vi "CRYReport Pic TX LIB.vi"(6 "Control Ref":refnum<k7>, 7 "sAction":string, 8 "nData":i32, 9 "sData":string, 10 "TXTextControl":refnum<k7>, 11 "cFrame":T1) -> (0 "nData_Out":i32, 1 "sData_Out":string, 3 "cFrame_Out":T1)   [LabVIEW 2013]
uses:
  CRYReport Global.vi
  CRYProject/CRYProject Editor Global.vi
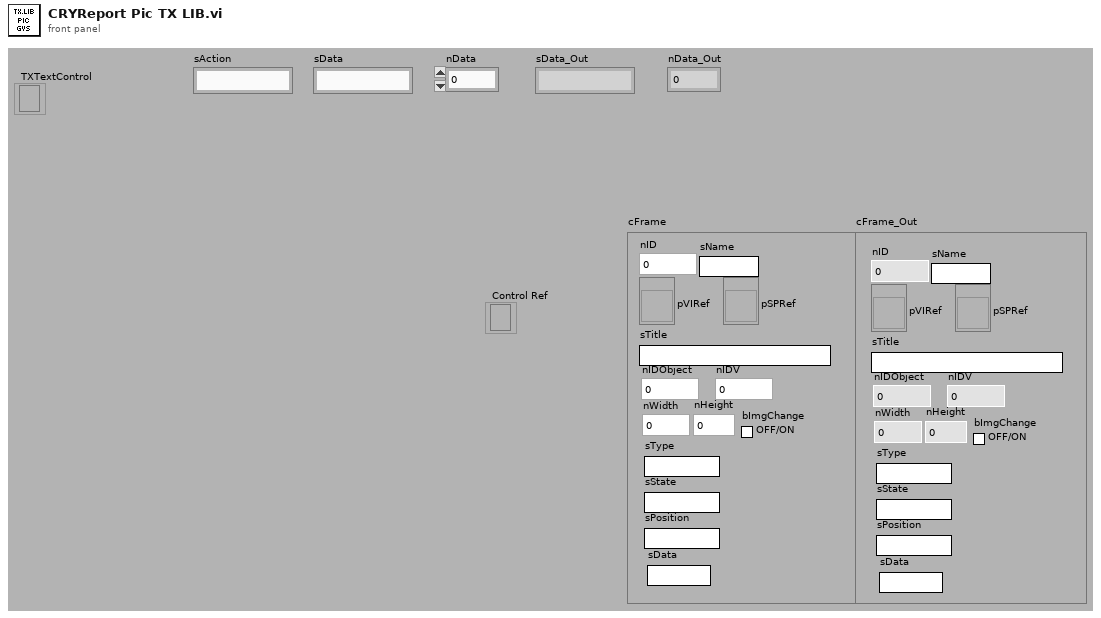
[diagram p1: front panel]
types:
  T1 = cluster{"nID":i16, "sName":string, "pVIRef":refnum<vi>, "pSPRef":refnum<vi>, "sTitle":string, "nIDObject":i16, "nIDV":i16, "nWidth":i16, "nHeight":i16, "bImgChange":bool, "sType":string, "sState":string, "sPosition":string, "sData":string}
  T2 = enum16{"open", "open or create", "create or replace", "create", "open (read only)"}
  T3 = typedef "CRYTS.ctl" = cluster{"No.TS":u16, "TS File Path":path, "TS Name":string, "EditStepName":string, "Steps":T4[], "New State":bool, "Change State":bool, "Flattened CurveLib Data":string, "Document Data":string, "EditStepNo":u16, "Operator Start File":string, "Sequence Type":string, "Sequence Language":string}
  T4 = typedef "CRYStep.ctl" = cluster{"No.VI":i32, "Category":string, "StepName":string, "Seq setup flattened":string, "Comment":string, "Steps config.":bool[], "Jump config":i32[], "Start":dbl, "Increment":dbl, "Name":string, "Unit":string, "Y data":u16, "Y prefix":string, "Y dB ref":dbl, "Y unit":string, "Repeat State Array":cluster{"Start":dbl, "Increment":dbl, "Count":i32, "Num":i32}[]}
  T5 = typedef "LVRectTypeDef.ctl" = cluster{"Left":i16, "Top":i16, "Right":i16, "Bottom":i16}
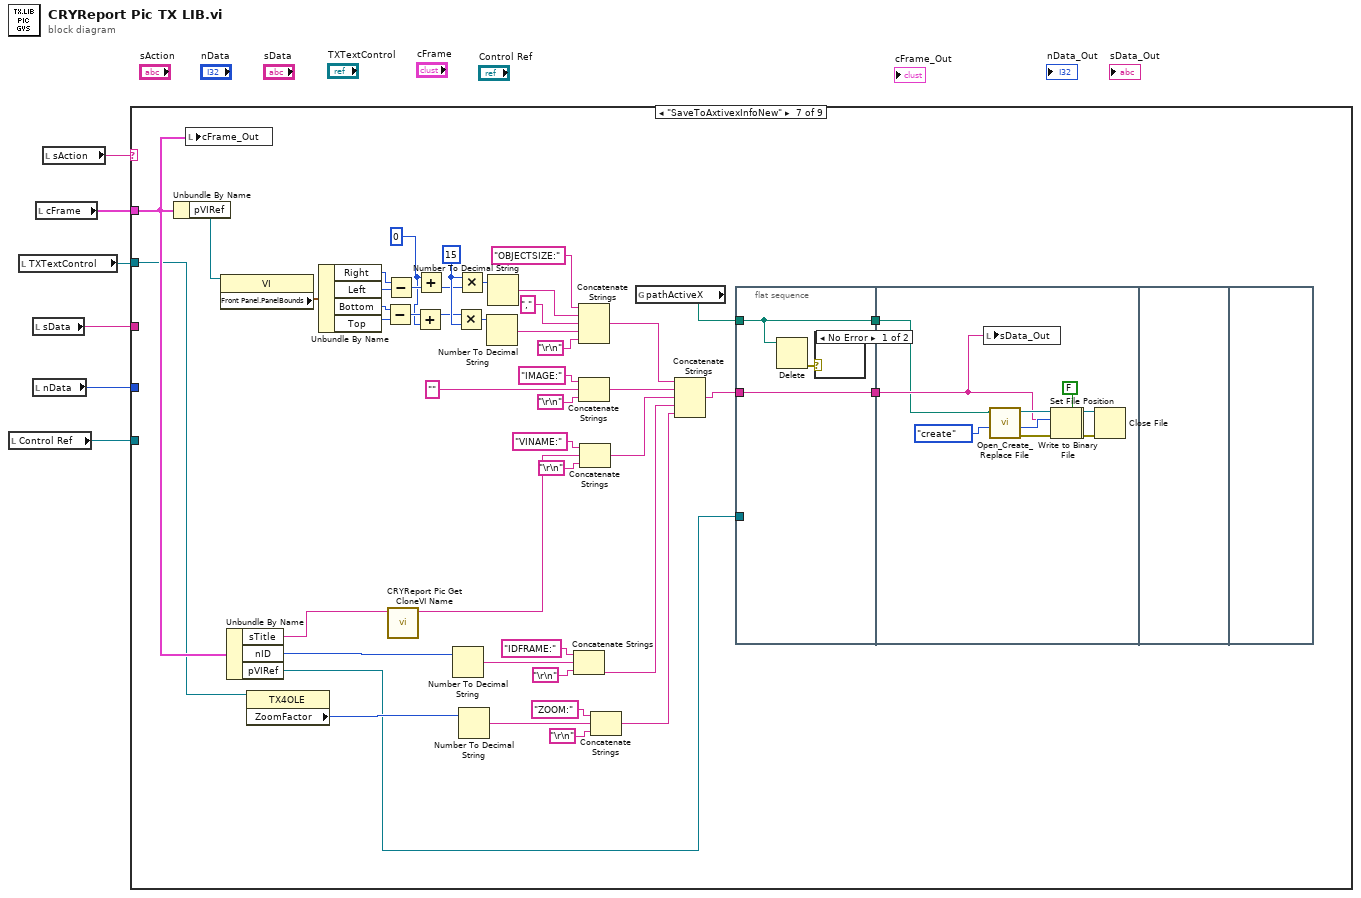
[diagram p0: block diagram]
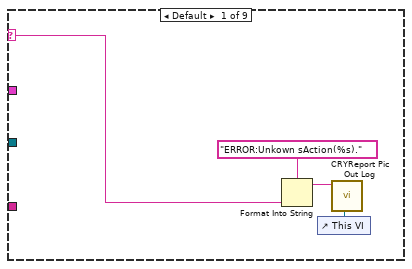
[diagram p2: hidden frame]
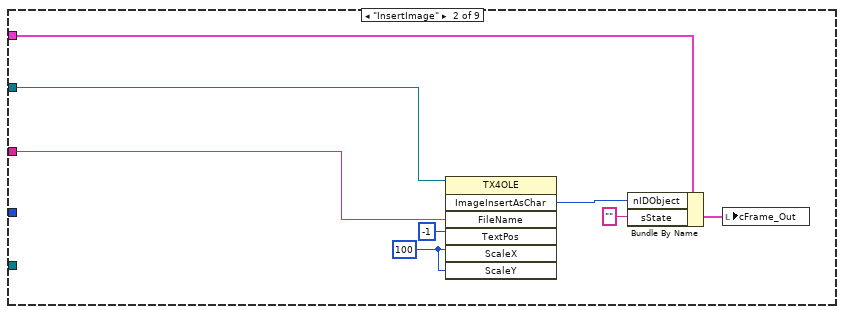
[diagram p3: hidden frame]
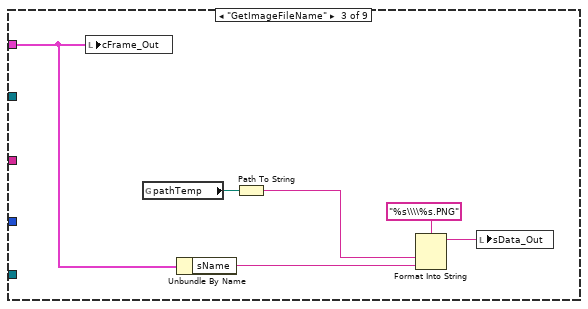
[diagram p4: hidden frame]
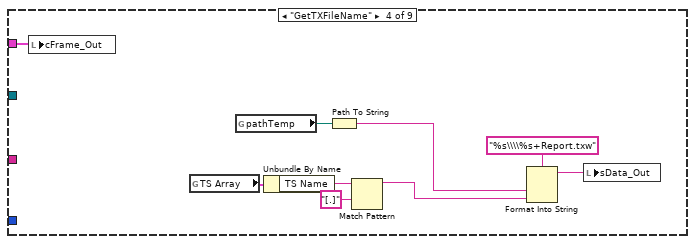
[diagram p5: hidden frame]
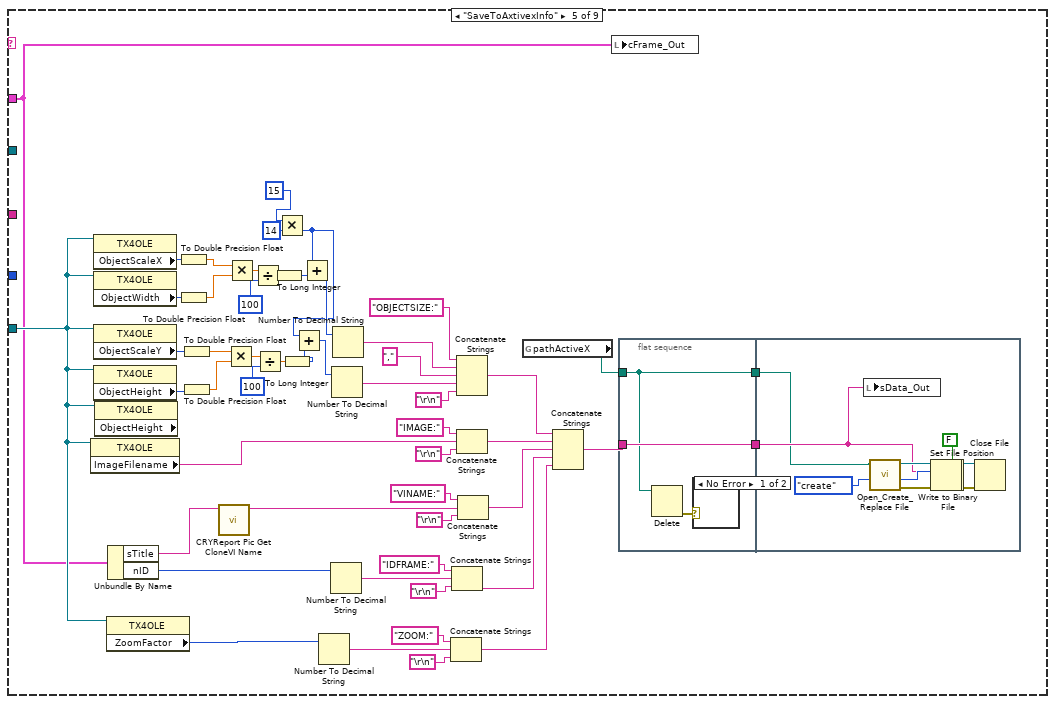
[diagram p6: hidden frame]
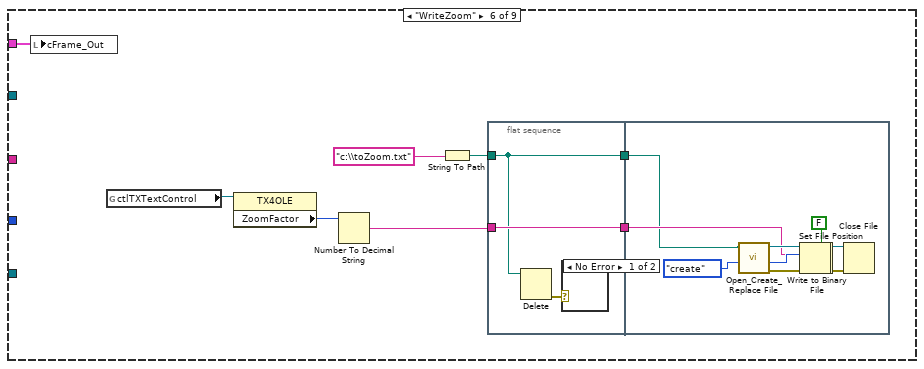
[diagram p8: hidden frame]
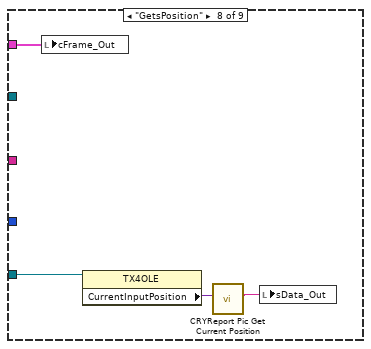
[diagram p11: hidden frame]
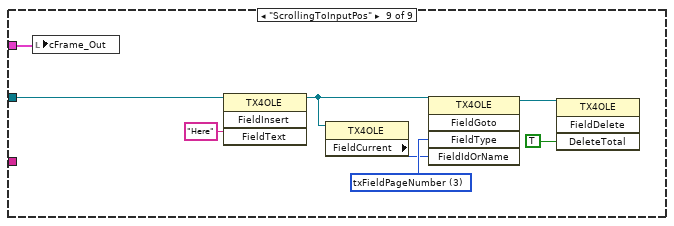
[diagram p12: hidden frame]
diagram:
  n1 = local read "Control Ref"() -> (w1:refnum<k7>)
  n2 = local read "TXTextControl"() -> (w2:refnum<k7>)
  n3 = local read "sData"() -> (w5:string)
  n4 = local read "nData"() -> (w4:i32)
  n5 = local read "cFrame"() -> (w3:T1)
  n6 = local read "sAction"() -> (w6:string)
  n7 = case shown="\"SaveToAxtivexInfoNew\"" w6 {
    selector: w6 -> [w8 _ _ _ _ _ _ _ _]
    tunnel: w5 -> [_ w11 _ _ _ _ _ _ _]
    tunnel: w4 -> [_ _ _ _ _ _ _ _ _]
    tunnel: w3 -> [_ w13 w19 w25 w40 w100 w147 w184 w186]
    tunnel: w2 -> [_ w12 _ _ _ _ w129 _ w187]
    tunnel: w1 -> [_ _ _ _ w44 _ _ w185 _]
    frame Default {
      n8 = Format Into String(format string="ERROR:Unkown sAction(%s).", w8) -> (resulting string=w7:string)  [unwired: 2 in, 1 out]
      n9 = control-ref of="This VI"() -> (w10:refnum<vi>)
      n10 = call "CRYReport Pic Out Log.vi"("vi reference"=w10, "sData"=w7) -> ()  [unwired: 10 in]
    }
    frame "InsertImage" {
      w17 = i16 100 ("ScaleX")
      n11 = invoke class="TX4OLE" method="ImageInsertAsChar"(reference=w12, "FileName"=w11, "TextPos"=-1, "ScaleX"=w17, "ScaleY"=w17) -> ("ImageInsertAsChar"=w16:i16)  [unwired: 2 in, 6 out]
      n12 = Bundle By Name(cluster=w13, "nIDObject"=w16, "sState"="") -> (w15:T1)
      n13 = local write "cFrame_Out"(w15) -> ()
    }
    frame "GetImageFileName" {
      n14 = local write "cFrame_Out"(w19) -> ()
      n15 = global read "CRYReport Global.vi" "pathTemp"() -> (w24:path)
      n16 = Unbundle By Name(w19) -> ("sName"=w21:string)
      n17 = Path To String(path=w24) -> (string=w22:string)
      n18 = Format Into String(format string="%s\\\\%s.PNG", w22, w21) -> (resulting string=w20:string)  [unwired: 2 in, 1 out]
      n19 = local write "sData_Out"(w20) -> ()
    }
    frame "GetTXFileName" {
      n20 = local write "cFrame_Out"(w25) -> ()
      n21 = global read "CRYProject Editor Global.vi" "TS Array"() -> (w32:T3)
      n22 = global read "CRYReport Global.vi" "pathTemp"() -> (w33:path)
      n23 = Unbundle By Name(w32) -> ("TS Name"=w31:string)
      n24 = Path To String(path=w33) -> (string=w28:string)
      n25 = Match Pattern(string=w31, regular expression="[.]") -> (before substring=w27:string)  [unwired: 1 in, 3 out]
      n26 = Format Into String(format string="%s\\\\%s+Report.txw", w28, w27) -> (resulting string=w26:string)  [unwired: 2 in, 1 out]
      n27 = local write "sData_Out"(w26) -> ()
    }
    frame "SaveToAxtivexInfo" {
      n28 = property class="TX4OLE"(reference=w44) -> ("ImageFilename"=w59:string)  [unwired: 1 in, 2 out]
      n29 = property class="TX4OLE"(reference=w44) -> ("ObjectScaleX"=w50:i16)  [unwired: 1 in, 2 out]
      n30 = property class="TX4OLE"(reference=w44) -> ("ObjectWidth"=w49:i16)  [unwired: 1 in, 2 out]
      n31 = property class="TX4OLE"(reference=w44) -> ("ObjectScaleY"=w67:i16)  [unwired: 1 in, 2 out]
      n32 = property class="TX4OLE"(reference=w44) -> ("ObjectHeight"=w66:i16)  [unwired: 1 in, 2 out]
      n33 = property class="TX4OLE" props=["ObjectHeight"](reference=w44) -> ()  [unwired: 1 in, 3 out]
      n34 = property class="TX4OLE"(reference=w44) -> ("ZoomFactor"=w43:i16)  [unwired: 1 in, 2 out]
      n35 = Unbundle By Name(w40) -> ("sTitle"=w42:string, "nID"=w55:i16)
      n36 = To Double Precision Float(number=w50) -> (double precision float=w68:dbl)
      n37 = To Double Precision Float(number=w49) -> (double precision float=w69:dbl)
      n38 = To Double Precision Float(number=w67) -> (double precision float=w65:dbl)
      n39 = To Double Precision Float(number=w66) -> (double precision float=w64:dbl)
      n40 = call "CRYReport Pic Get CloneVI Name.vi"("sTitle"=w42) -> ("sVIName_Out"=w41:string)  [unwired: 10 in]
      n41 = Multiply(x=w65, y=w64) -> (x*y=w73:dbl)
      n42 = Multiply(x=w68, y=w69) -> (x*y=w76:dbl)
      n43 = Divide(x=w76, y=i16 100) -> (x/y=w72:dbl)
      n44 = Divide(x=w73, y=i16 100) -> (x/y=w70:dbl)
      n45 = To Long Integer(number=w72) -> (32bit integer=w71:i32)
      n46 = Multiply(x=15, y=14 ("x")) -> (x*y=w34:i32)
      n47 = To Long Integer(number=w70) -> (32bit integer=w37:i32)
      n48 = Add(x=w34, y=w37) -> (x+y=w36:i32)
      n49 = Add(x=w34, y=w71) -> (x+y=w39:i32)
      n50 = Number To Decimal String(number=w43) -> (decimal integer string=w45:string)  [unwired: 1 in]
      n51 = Number To Decimal String(number=w55) -> (decimal integer string=w79:string)  [unwired: 1 in]
      n52 = Number To Decimal String(number=w36) -> (decimal integer string=w85:string)  [unwired: 1 in]
      n53 = Number To Decimal String(number=w39) -> (decimal integer string=w57:string)  [unwired: 1 in]
      n54 = Concatenate Strings("ZOOM:" ("string"), w45, "\r\n") -> (w46:string)
      n55 = Concatenate Strings("IDFRAME:" ("string"), w79, "\r\n") -> (w63:string)
      n56 = Concatenate Strings("OBJECTSIZE:" ("string"), w57, "," ("string"), w85, "\r\n") -> (w77:string)
      n57 = Concatenate Strings("IMAGE:" ("string"), w59, "\r\n") -> (w78:string)
      n58 = Concatenate Strings("VINAME:" ("string"), w41, "\r\n") -> (w60:string)
      n59 = global read "CRYReport Global.vi" "pathActiveX"() -> (w51:path)
      n60 = Concatenate Strings(w77, w78, w60, w63, w46) -> (w52:string)
      n61 = local write "cFrame_Out"(w40) -> ()
      n62 = flat-sequence {
        tunnel: w52 -> [w88]
        tunnel: [w88] -> w54
        tunnel: w51 -> [w87]
        tunnel: [w87] -> w53
        tunnel: w54 -> [w90]
        tunnel: w53 -> [w89]
        frame #0 {
          n63 = Delete(path (use dialog)=w87) -> (error out=w86:errorcluster)  [unwired: 4 in, 2 out]
          n64 = case shown="No Error" w86 {
            frame No Error {
            }
            frame Error {
            }
          }
        }
        frame #1 {
          n65 = local write "sData_Out"(w90) -> ()
          n66 = call <vilib>:"Open_Create_Replace File.vi"("function (open:0)"=T2."create", "file path"=w89) -> ("error out"=w98:errorcluster, "file size (bytes)"=w96:i32, "refnum"=w97:refnum<file>)  [unwired: 6 in, 1 out]
          n67 = Set File Position(offset (in bytes) (0)=w96, refnum=w97, error in=w98) -> (refnum out=w93:refnum<file>, error out=w92:errorcluster)  [unwired: 1 in]
          n68 = Write to Binary File(file (use dialog)=w93, data=w90, error in=w92, 5:FALSE ("prepend array or string size? (T)")) -> (refnum out=w94:refnum<file>, error out=w95:errorcluster)  [unwired: 2 in, 1 out]
          n69 = Close File(refnum=w94, error in=w95) -> ()  [unwired: 2 out]
        }
      }
    }
    frame "WriteZoom" {
      n70 = local write "cFrame_Out"(w100) -> ()
      n71 = global read "CRYReport Global.vi" "ctlTXTextControl"() -> (w101:refnum<k7>)
      n72 = property class="TX4OLE"(reference=w101) -> ("ZoomFactor"=w103:i16)  [unwired: 1 in, 2 out]
      n73 = Number To Decimal String(number=w103) -> (decimal integer string=w102:string)  [unwired: 1 in]
      n74 = String To Path(string="c:\\toZoom.txt") -> (path=w105:path)
      n75 = flat-sequence {
        tunnel: w102 -> [w110]
        tunnel: [w110] -> w107
        tunnel: w105 -> [w109]
        tunnel: [w109] -> w106
        tunnel: w107 -> [w112]
        tunnel: w106 -> [w111]
        frame #0 {
          n76 = Delete(path (use dialog)=w109) -> (error out=w108:errorcluster)  [unwired: 4 in, 2 out]
          n77 = case shown="No Error" w108 {
            frame No Error {
            }
            frame Error {
            }
          }
        }
        frame #1 {
          n78 = call <vilib>:"Open_Create_Replace File.vi"("function (open:0)"=T2."create", "file path"=w111) -> ("error out"=w120:errorcluster, "file size (bytes)"=w118:i32, "refnum"=w119:refnum<file>)  [unwired: 6 in, 1 out]
          n79 = Set File Position(offset (in bytes) (0)=w118, refnum=w119, error in=w120) -> (refnum out=w115:refnum<file>, error out=w114:errorcluster)  [unwired: 1 in]
          n80 = Write to Binary File(file (use dialog)=w115, data=w112, error in=w114, 5:FALSE ("prepend array or string size? (T)")) -> (refnum out=w116:refnum<file>, error out=w117:errorcluster)  [unwired: 2 in, 1 out]
          n81 = Close File(refnum=w116, error in=w117) -> ()  [unwired: 2 out]
        }
      }
    }
    frame "SaveToAxtivexInfoNew" {
      w122 = i16 0 ("x")
      w135 = i16 15 ("x")
      n82 = Unbundle By Name(w147) -> ("pVIRef"=w146:refnum<vi>)
      n83 = local write "cFrame_Out"(w147) -> ()
      n84 = property class="VI"(reference=w146) -> ("Front Panel.PanelBounds"=w145:T5)  [unwired: 1 in, 2 out]
      n85 = Unbundle By Name(w147) -> ("sTitle"=w125:string, "nID"=w151:i16, "pVIRef"=w127:refnum<vi>)
      n86 = property class="TX4OLE"(reference=w129) -> ("ZoomFactor"=w131:i16)  [unwired: 1 in, 2 out]
      n87 = Unbundle By Name(w145) -> ("Right"=w143:i16, "Left"=w144:i16, "Bottom"=w142:i16, "Top"=w141:i16)
      n88 = Subtract(x=w142, y=w141) -> (x-y=w137:i16)
      n89 = Subtract(x=w143, y=w144) -> (x-y=w139:i16)
      n90 = call "CRYReport Pic Get CloneVI Name.vi"("sTitle"=w125) -> ("sVIName_Out"=w126:string)  [unwired: 10 in]
      n91 = Add(x=w137, y=w122) -> (x+y=w124:i16)
      n92 = Add(x=w122, y=w139) -> (x+y=w123:i16)
      n93 = Number To Decimal String(number=w151) -> (decimal integer string=w161:string)  [unwired: 1 in]
      n94 = Multiply(x=w124, y=w135) -> (x*y=w136:i16)
      n95 = Multiply(x=w135, y=w123) -> (x*y=w138:i16)
      n96 = Number To Decimal String(number=w131) -> (decimal integer string=w132:string)  [unwired: 1 in]
      n97 = Number To Decimal String(number=w136) -> (decimal integer string=w167:string)  [unwired: 1 in]
      n98 = Number To Decimal String(number=w138) -> (decimal integer string=w153:string)  [unwired: 1 in]
      n99 = Concatenate Strings("IDFRAME:" ("string"), w161, "\r\n") -> (w158:string)
      n100 = Concatenate Strings("OBJECTSIZE:" ("string"), w153, "," ("string"), w167, "\r\n") -> (w159:string)
      n101 = Concatenate Strings("IMAGE:" ("string"), "" ("string"), "\r\n") -> (w160:string)
      n102 = Concatenate Strings("VINAME:" ("string"), w126, "\r\n") -> (w155:string)
      n103 = Concatenate Strings("ZOOM:" ("string"), w132, "\r\n") -> (w130:string)
      n104 = global read "CRYReport Global.vi" "pathActiveX"() -> (w140:path)
      n105 = Concatenate Strings(w159, w160, w155, w158, w130) -> (w128:string)
      n106 = flat-sequence {
        tunnel: w128 -> [w170]
        tunnel: [w170] -> w150
        tunnel: w140 -> [w169]
        tunnel: [w169] -> w149
        tunnel: w127 -> [_]
        tunnel: w150 -> [w172]
        tunnel: w149 -> [w171]
        frame #0 {
          n107 = Delete(path (use dialog)=w169) -> (error out=w168:errorcluster)  [unwired: 4 in, 2 out]
          n108 = case shown="No Error" w168 {
            frame No Error {
            }
            frame Error {
            }
          }
        }
        frame #1 {
          n109 = local write "sData_Out"(w172) -> ()
          n110 = call <vilib>:"Open_Create_Replace File.vi"("function (open:0)"=T2."create", "file path"=w171) -> ("error out"=w180:errorcluster, "file size (bytes)"=w178:i32, "refnum"=w179:refnum<file>)  [unwired: 6 in, 1 out]
          n111 = Set File Position(offset (in bytes) (0)=w178, refnum=w179, error in=w180) -> (refnum out=w175:refnum<file>, error out=w174:errorcluster)  [unwired: 1 in]
          n112 = Write to Binary File(file (use dialog)=w175, data=w172, error in=w174, 5:FALSE ("prepend array or string size? (T)")) -> (refnum out=w176:refnum<file>, error out=w177:errorcluster)  [unwired: 2 in, 1 out]
          n113 = Close File(refnum=w176, error in=w177) -> ()  [unwired: 2 out]
        }
        frame #2 {
        }
        frame #3 {
        }
      }
    }
    frame "GetsPosition" {
      n114 = local write "cFrame_Out"(w184) -> ()
      n115 = property class="TX4OLE"(reference=w185) -> ("CurrentInputPosition"=w183:variant)  [unwired: 1 in, 2 out]
      n116 = call "CRYReport Pic Get Current Position.vi"("CurrentInputPosition"=w183) -> ("sData_Out"=w182:string)  [unwired: 9 in, 1 out]
      n117 = local write "sData_Out"(w182) -> ()
    }
    frame "ScrollingToInputPos" {
      w192 = 3 items=["txFieldStandard", "txFieldExternalLink", "txFieldInternalLink", "txFieldPageNumber", "txFieldLinkTarget", "txFieldHighlight", "txFieldTopic", "txFieldMSWord", "txFieldHighEdit"] ("FieldType")
      n118 = local write "cFrame_Out"(w186) -> ()
      n119 = invoke class="TX4OLE" method="FieldInsert"(reference=w187, "FieldText"="Here") -> (reference out=w191:refnum<k7>)  [unwired: 2 in, 3 out]
      n120 = property class="TX4OLE"(reference=w191) -> ("FieldCurrent"=w190:i16)  [unwired: 1 in, 2 out]
      n121 = invoke class="TX4OLE" method="FieldGoto"(reference=w191, "FieldType"=w192, "FieldIdOrName"=w190) -> (reference out=w189:refnum<k7>)  [unwired: 2 in, 4 out]
      n122 = invoke class="TX4OLE" method="FieldDelete"(reference=w189, "DeleteTotal"=TRUE) -> ()  [unwired: 2 in, 4 out]
    }
  }
